vi "GetPathCost.vi"(1 "Path Cost Weights":T1={"Length Weight"=1.0, "Angle Weight"=0.0, "Angle Error Weight"=1000.0, "Angle Error Threshold"=0.314, "Per Move Penalty"=0.05, "Closeness Weight"=100.0, "Too Short Penalty"=100.0, "Too Short Threshold"=1.5}, 2 "Path":T2) -> (0 "Cost":dbl)   [LabVIEW 2015, in "Navigation2017.lvlib" / "Navigation2017-SubVIs.lvlib"]
uses:
  Navigation2017-SubVIs.lvlib
  Path.ctl
  Move.ctl
  PathCostWeights.ctl
  Navigation2017.lvlib
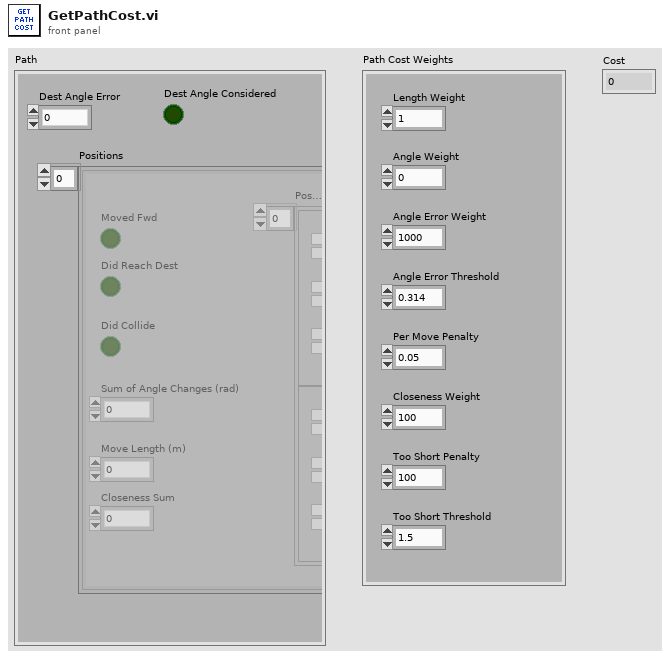
[diagram p1: front panel]
types:
  T1 = typedef "Navigation2017.lvlib/PathCostWeights.ctl" = cluster{"Length Weight":dbl, "Angle Weight":dbl, "Angle Error Weight":dbl, "Angle Error Threshold":dbl, "Per Move Penalty":dbl, "Closeness Weight":dbl, "Too Short Penalty":dbl, "Too Short Threshold":dbl}
  T2 = typedef "Navigation2017.lvlib/Path.ctl" = cluster{"Dest Angle Error":dbl, "Dest Angle Considered":bool, "Positions":T3[]}
  T3 = typedef "Navigation2017.lvlib/Move.ctl" = cluster{"Did Reach Dest":bool, "Did Collide":bool, "Sum of Angle Changes (rad)":dbl, "Move Length (m)":dbl, "Closeness Sum":dbl, "Positions Along Move":cluster{"x":dbl, "y":dbl, "angle":dbl}[], "Moved Fwd":bool}
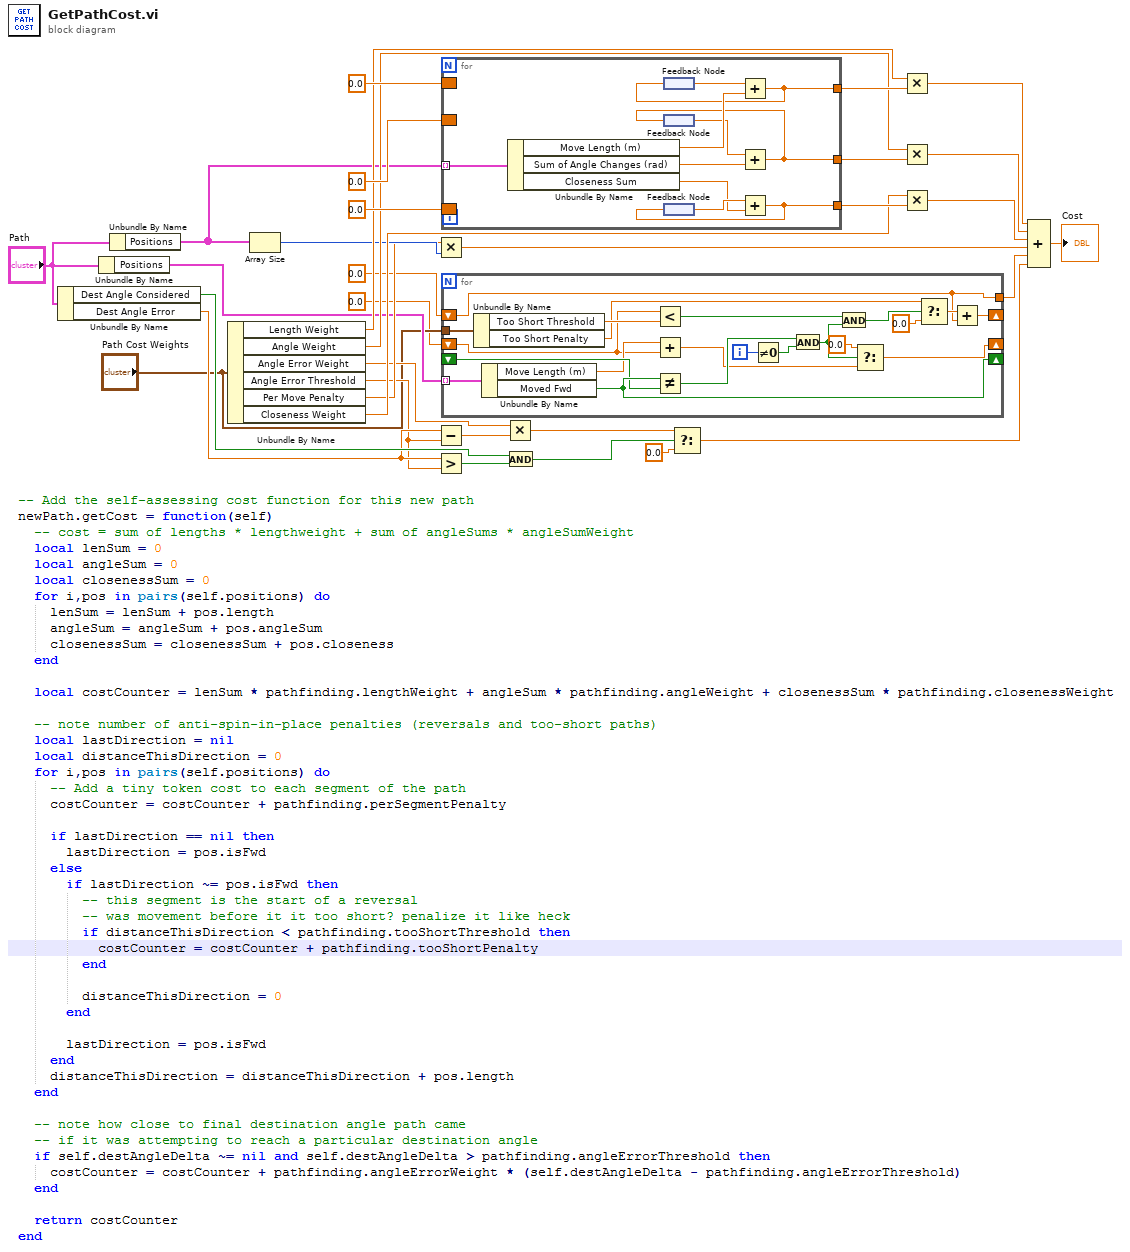
[diagram p0: block diagram]
diagram:
  n1 = Unbundle By Name("Path") -> ("Dest Angle Considered"=w16:bool, "Dest Angle Error"=w12:dbl)
  n2 = Unbundle By Name("Path") -> ("Positions"=w5:T3[])
  n3 = Unbundle By Name("Path") -> ("Positions"=w20:T3[])
  n4 = Unbundle By Name("Path Cost Weights") -> ("Length Weight"=w28:dbl, "Angle Weight"=w26:dbl, "Angle Error Weight"=w14:dbl, "Angle Error Threshold"=w11:dbl, "Per Move Penalty"=w18:dbl, "Closeness Weight"=w21:dbl)
  n5 = Array Size(array=w20) -> (size(s)=w19:i32)
  n6 = Multiply(x=w18, y=w19) -> (x*y=w17:dbl)
  n7 = Subtract(x=w12, y=w11) -> (x-y=w13:dbl)
  n8 = Greater?(x=w12, y=w11) -> (0:w15:bool)
  n9 = for {
    tunnel: w20 -> [w34] mode=indexing
    border: 0.0 -> [_]
    border: 0.0 -> [_]
    border: 0.0 -> [_]
    tunnel: [w37] -> w29
    tunnel: [w36] -> w25
    tunnel: [w35] -> w23
    n10 = Unbundle By Name(w34) -> ("Move Length (m)"=w43:dbl, "Sum of Angle Changes (rad)"=w40:dbl, "Closeness Sum"=w38:dbl)
    n11 = feedback #1() -> (w42:dbl)
    n12 = feedback #2() -> (w41:dbl)
    n13 = feedback #3() -> (w39:dbl)
    n14 = Add(x=w42, y=w43) -> (x+y=w37:dbl)
    n15 = feedback-in #1(w37) -> ()
    n16 = Add(x=w41, y=w40) -> (x+y=w36:dbl)
    n17 = feedback-in #2(w36) -> ()
    n18 = Add(x=w39, y=w38) -> (x+y=w35:dbl)
    n19 = feedback-in #3(w35) -> ()
  }
  n20 = for {
    tunnel: w5 -> [w64] mode=indexing
    shift-right: [w63] -> _
    shift-left: _ -> [w62]
    tunnel: "Path Cost Weights" -> [w58]
    tunnel: [w53] -> w1
    shift-right: [w52] -> _
    shift-left: 0.0 -> [w53]
    shift-right: [w49] -> _
    shift-left: 0.0 -> [w44]
    i -> [w59]
    n21 = Unbundle By Name(w58) -> ("Too Short Threshold"=w57:dbl, "Too Short Penalty"=w56:dbl)
    n22 = Unbundle By Name(w64) -> ("Move Length (m)"=w45:dbl, "Moved Fwd"=w63:bool)
    n23 = Less?(x=w44, y=w57) -> (x < y?=w50:bool)
    n24 = Add(x=w45, y=w44) -> (x+y=w46:dbl)
    n25 = Not Equal?(x=w63, y=w62) -> (x != y?=w61:bool)
    n26 = Not Equal To 0?(x=w59) -> (x != 0?=w60:bool)
    n27 = And(x=w61, y=w60) -> (x .and. y?=w48:bool)
    n28 = And(x=w50, y=w48) -> (x .and. y?=w51:bool)
    n29 = Select(t=0.0, s=w48, f=w46) -> (s? t:f=w49:dbl)
    n30 = Select(t=w56, s=w51, f=0.0) -> (s? t:f=w54:dbl)
    n31 = Add(x=w54, y=w53) -> (x+y=w52:dbl)
  }
  n32 = Multiply(x=w14, y=w13) -> (x*y=w10:dbl)
  n33 = And(x=w16, y=w15) -> (x .and. y?=w9:bool)
  n34 = Select(t=w10, s=w9, f=0.0) -> (s? t:f=w7:dbl)
  n35 = Multiply(x=w28, y=w29) -> (x*y=w27:dbl)
  n36 = Multiply(x=w26, y=w25) -> (x*y=w24:dbl)
  n37 = Multiply(x=w21, y=w23) -> (x*y=w22:dbl)
  n38 = Compound Arithmetic op=ADD(w27, w24, w22, w17, w1, w7) -> (→"Cost":dbl)
